vi "Helper - Add Randomness.vi"(8 "Amplitude (1)":dbl=1.0, 11 "Numeric in":dbl) -> (3 "Numeric out":dbl)   [LabVIEW 2011]
doc: "Adds random noise to the input signal, with the noise ranging from -amplitude to +amplitude. If no input signal is provided, returns just the noise."
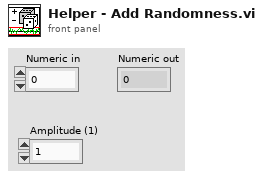
[diagram p1: front panel]
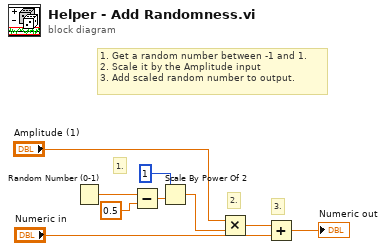
[diagram p0: block diagram]
diagram:
  # "3."
  # "1. Get a random number between -1 and 1.\n2. Scale it by the Amplitude input\n3. Add scaled random number to output."
  # "2."
  # "1."
  n1 = Random Number (0-1)() -> (number: 0 to 1=w7:dbl)
  n2 = Subtract(x=w7, y=0.5) -> (x-y=w6:dbl)
  n3 = Scale By Power Of 2(n=1, x=w6) -> (x*2^n=w2:dbl)
  n4 = Multiply(x="Amplitude (1)", y=w2) -> (x*y=w8:dbl)
  n5 = Add(x=w8, y="Numeric in") -> (x+y=→"Numeric out":dbl)
